vi "create_corewebview_env.vi"(8 "error in":errorcluster) -> (0 "error out":errorcluster, 3 "Environment":refnum<k24>)   [LabVIEW 2020, in "simple_html_chat_ui.lvclass"]
uses:
  simple_html_chat_ui.lvclass
  D:/Personal/LabVIEW LLMs/user_interfaces/simple_html_chat_ui/assembly_support/Microsoft.Web.WebView2.Core.dll
  assembly_support/Microsoft.Web.WebView2.Core.dll
  <vilib>/Utility/sysdir.llb/System Directory Type.ctl
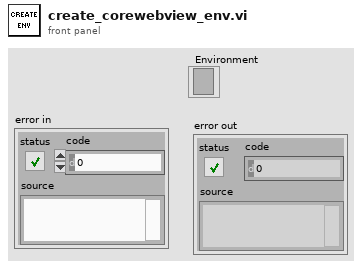
[diagram p1: front panel]
types:
  T1 = typedef "System Directory Type.ctl" = i32
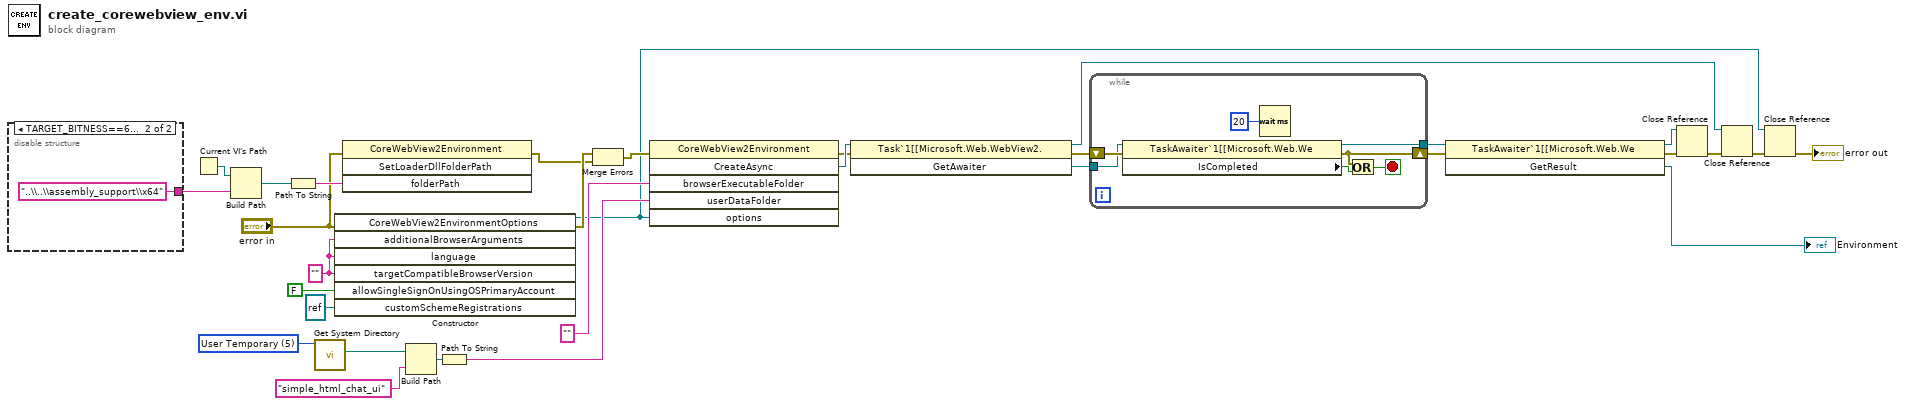
[diagram p0: block diagram]
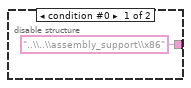
[diagram p2: hidden frame]
diagram:
  w13 = "" ("additionalBrowserArguments")
  w30 = T1 5 items=["User Home"=0, "User Desktop"=1, "User Documents"=2, "User Application Data"=3, "User Preferences"=4, "User Temporary"=5, "Public Documents"=6, "Public Application Data"=7, "Public Preferences"=8, "Public Cache"=13, "System Core Libraries"=9, "System Installed Libraries"=10, "Application Files"=11, "Boot Volume Root"=12] ("system directory type")
  n1 = disable-structure shown="TARGET_BITNESS==64" {
    disable-tunnel: ["..\\..\\assembly_support\\x86" "..\\..\\assembly_support\\x64"] -> w26
    frame condition #0 {
    }
    frame condition #1 (active) {
    }
  }
  n2 = Current VI's Path() -> (path=w25:path)
  n3 = Build Path(base path=w25, name or relative path=w26) -> (appended path=w24:path)
  n4 = Path To String(path=w24) -> (string=w16:string)
  n5 = call <vilib>:"Get System Directory.vi"("system directory type"=w30) -> ("system directory"=w29:path)  [unwired: 10 in]
  n6 = constructor class="CoreWebView2EnvironmentOptions"(error in="error in", "additionalBrowserArguments"=w13, "language"=w13, "targetCompatibleBrowserVersion"=w13, "allowSingleSignOnUsingOSPrimaryAccount"=FALSE, "customSchemeRegistrations"=refnum<k24> refnum) -> (reference out=w1:refnum<k24>, error out=w18:errorcluster)  [unwired: 2 in, 6 out]
  n7 = invoke class="CoreWebView2Environment" method="SetLoaderDllFolderPath"(error in="error in", "folderPath"=w16) -> (error out=w7:errorcluster)  [unwired: 2 in, 3 out]
  n8 = Build Path(base path=w29, name or relative path="simple_html_chat_ui") -> (appended path=w27:path)
  n9 = Path To String(path=w27) -> (string=w17:string)
  n10 = Merge Errors(w18, w7) -> (w8:errorcluster)
  n11 = invoke class="CoreWebView2Environment" method="CreateAsync"(error in=w8, "browserExecutableFolder"="", "userDataFolder"=w17, "options"=w1) -> (error out=w14:errorcluster, "CreateAsync"=w23:refnum<k24>)  [unwired: 2 in, 4 out]
  n12 = invoke class="Task`1[[Microsoft.Web.WebView2." method="GetAwaiter"(reference=w23, error in=w14) -> (reference out=w4:refnum<k24>, error out=w22:errorcluster, "GetAwaiter"=w15:refnum<k24>)  [unwired: 1 in]
  n13 = while {
    tunnel: w15 -> [w39]
    shift-right: [w34] -> w19
    shift-left: w22 -> [w40]
    tunnel: [w36] -> w21
    stop <- w35 stop-if-true
    n14 = property class="TaskAwaiter`1[[Microsoft.Web.We"(reference=w39, error in=w40) -> (reference out=w36:refnum<k24>, error out=w34:errorcluster, "IsCompleted"=w37:bool)
    n15 = Wait (ms)(milliseconds to wait=u32 20 ("millisecond multiple")) -> ()  [unwired: 1 out]
    n16 = Or(x=w34, y=w37) -> (x .or. y?=w35:bool)
  }
  n17 = invoke class="TaskAwaiter`1[[Microsoft.Web.We" method="GetResult"(reference=w21, error in=w19) -> (reference out=w20:refnum<k24>, error out=w11:errorcluster, "GetResult"=→"Environment":refnum<k24>)  [unwired: 1 in]
  n18 = Close Reference(reference=w20, error in (no error)=w11) -> (error out=w5:errorcluster)
  n19 = Close Reference(reference=w4, error in (no error)=w5) -> (error out=w3:errorcluster)
  n20 = Close Reference(reference=w1, error in (no error)=w3) -> (error out=→"error out":errorcluster)
